vi "enum_to_single.vi"(11 "hi":u8) -> (3 "Numeric":sgl format="%#4_6g")   [LabVIEW 2017]
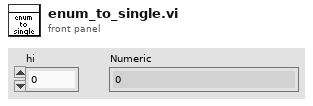
[diagram p1: front panel]
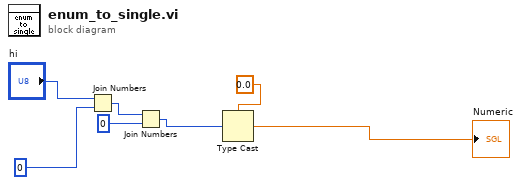
[diagram p0: block diagram]
diagram:
  n1 = Join Numbers(hi="hi", lo=u8 0) -> ((hi.lo)=w1:u16)
  n2 = Join Numbers(hi=w1, lo=u16 0) -> ((hi.lo)=w5:u32)
  n3 = Type Cast(type=sgl 0.0, x=w5) -> (*(type *) &x=→"Numeric":sgl)
